vi "DataLoggingSessionStop Event Callback.vi"(4 "Stop Event":refnum<user-event>, 5 "Event Data":cluster{"sender":refnum<k24>, "e":refnum<k24>}, 6 "Data Logging Manager Ref":T1, 7 "Event Common Data":T2) -> ()   [LabVIEW 2020, in "NI_VS Data Logging API.lvlib"]
uses:
  <vilib>/NI VeriStand/Execution/DataLogging/NI_VS Data Logging API.lvlib
  <vilib>/NI VeriStand/Execution/DataLogging/IDataLogging Ref.ctl
  NationalInstruments.VeriStand.ClientAPI
  <vilib>/NI VeriStand/Execution/DataLogging/Data Logging Session Stop Event Data.ctl
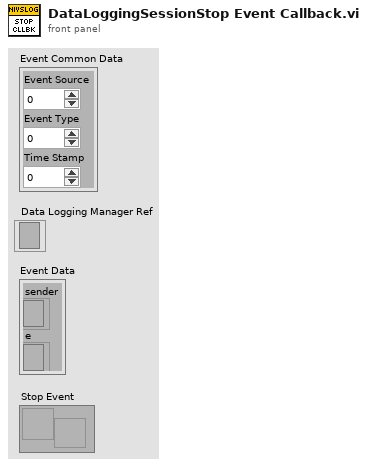
[diagram p1: front panel]
types:
  T1 = typedef "NI_VS Data Logging API.lvlib/IDataLogging Ref.ctl" = refnum<k24>
  T2 = cluster{"Event Source":i32, "Event Type":u32, "Time Stamp":u32}
  T3 = typedef "NI_VS Data Logging API.lvlib/Data Logging Session Stop Event Data.ctl" = cluster{"Session Name":string, "Log File Paths":path[]}
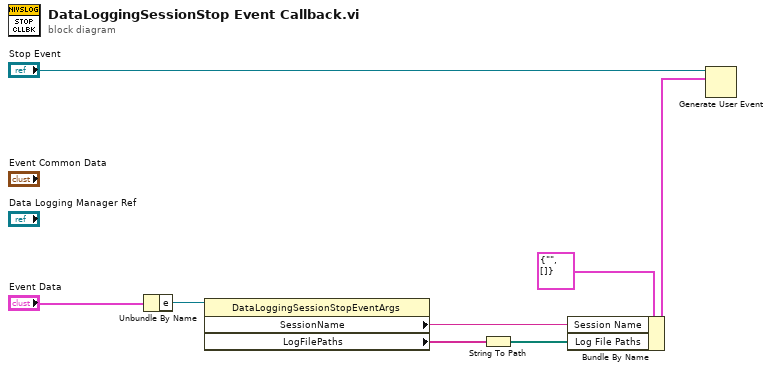
[diagram p0: block diagram]
diagram:
  n1 = Unbundle By Name("Event Data") -> ("e"=w8:refnum<k24>)
  n2 = property class="DataLoggingSessionStopEventArgs"(reference=w8) -> ("SessionName"=w7:string, "LogFilePaths"=w2:string[])  [unwired: 1 in, 2 out]
  n3 = String To Path(string=w2) -> (path=w1:path[])
  n4 = Bundle By Name(cluster=T3 {"Session Name"="", "Log File Paths"=[]} ("event data"), "Session Name"=w7, "Log File Paths"=w1) -> (w4:T3)
  n5 = Generate User Event(user event="Stop Event", event data cluster=w4) -> ()  [unwired: 2 in, 2 out]
